vi "Register for Manager Subpanel Events.vi"(8 "error in (no error)":errorcluster, 11 "CIF_Manager_UI in":refnum<class "CIF_Manager_UI.lvclass">) -> (0 "error out":errorcluster, 3 "Event Registration Refnum":refnum<event-registration>)   [LabVIEW 2021, in "CIF_Manager_UI.lvclass"]
uses:
  CIF_Manager_UI.lvclass
  C:/Program Files/National Instruments/LabVIEW 2021/vi.lib/CIF Foundation/CIF Core/CIFUI/CIF_UI.lvclass
  <vilib>/CIF Foundation/CIF Core/CIFUI/Typedef/New Connection Plugin Event Data.ctl
  CIFPluginManager/typedef/New Connection Event Data.ctl
  <vilib>/gRPC/LabVIEW gRPC Library/Shared/grpcId.ctl
  CIF_Manager_UI.lvclass/CIF_Manager_UI.ctl
  <vilib>/CIF Foundation/CIF Core/CIFUI/CIF_UI.lvclass/CIF_UI.ctl
  <vilib>/CIF Foundation/CIF Core/CIFUI/Accessors/Read Subpanel Events.vi
  <vilib>/CIF Foundation/CIF Core/CIFUI/CIF_UI.lvclass
  <vilib>/gRPC/LabVIEW gRPC Library/grpc-lvsupport-release.lvlib
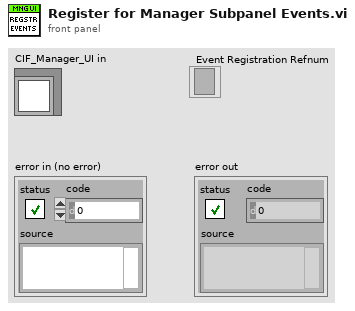
[diagram p1: front panel]
types:
  T1 = typedef "CIF_UI.lvclass/SubPanel Events.ctl" = cluster{"Clear Local Error":refnum<user-event>, "Shutdown":refnum<user-event>, "Plugin Connection":refnum<user-event>}
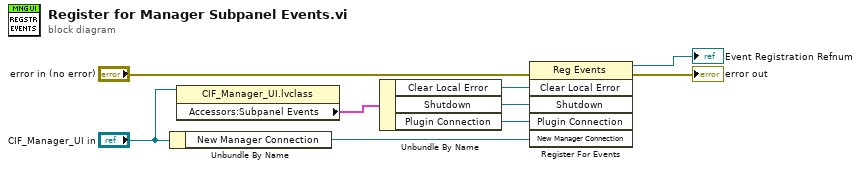
[diagram p0: block diagram]
diagram:
  n1 = Unbundle By Name("CIF_Manager_UI in") -> ("New Manager Connection"=w1:refnum<user-event>)
  n2 = property class="CIF_Manager_UI.lvclass"(reference="CIF_Manager_UI in") -> ("Accessors:Subpanel Events"=w4:T1)  [unwired: 1 in, 2 out]
  n3 = Unbundle By Name(w4) -> ("Clear Local Error"=w9:refnum<user-event>, "Shutdown"=w8:refnum<user-event>, "Plugin Connection"=w7:refnum<user-event>)
  n4 = register-events(error in="error in (no error)", w9, w8, w7, w1) -> (reference out=→"Event Registration Refnum":refnum<event-registration>, error out=→"error out":errorcluster)  [unwired: 1 in]
